vi "ApagarRIGOLDP832.vi"(8 "error in (no error)":errorcluster, 11 "VISA resource name":refnum<visa-resource-name>) -> (0 "error out":errorcluster, 3 "VISA resource name out":refnum<visa-resource-name>)   [LabVIEW 2019]
uses:
  Rigol DP832/DP832_Control Channels.ctl
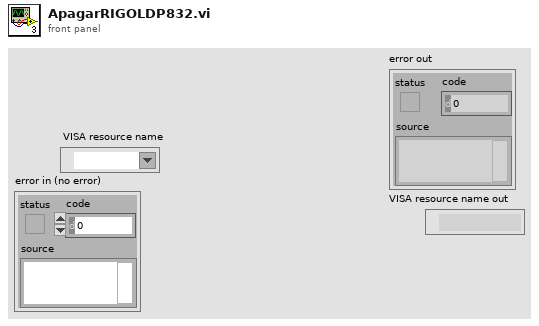
[diagram p1: front panel]
types:
  T1 = typedef "DP832_Control Channels.ctl" = i32
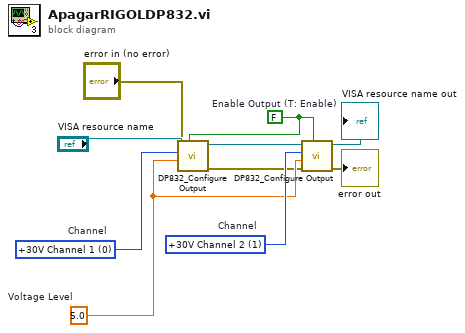
[diagram p0: block diagram]
diagram:
  w5 = 5.0  # Voltage Level
  w6 = FALSE  # Enable Output (T: Enable)
  w7 = T1 1 items=["+30V Channel 1", "+30V Channel 2", "+5V Channel 3"]  # Channel
  w9 = T1 0 items=["+30V Channel 1", "+30V Channel 2", "+5V Channel 3"]  # Channel
  n1 = call "DP832_Configure Output.vi"("Enable Output (T: Enable)"=w6, "error in (no error)"="error in (no error)", "Voltage Level"=w5, "Channel"=w9, "VISA resource name"="VISA resource name") -> ("error out"=w4:errorcluster, "VISA resource name out"=w8:refnum<visa-resource-name>)  [unwired: 5 in]
  n2 = call "DP832_Configure Output.vi"("Enable Output (T: Enable)"=w6, "error in (no error)"=w4, "Voltage Level"=w5, "Channel"=w7, "VISA resource name"=w8) -> ("error out"=→"error out":errorcluster, "VISA resource name out"=→"VISA resource name out":refnum<visa-resource-name>)  [unwired: 5 in]
